vi "Find One Cycle.vi"(11 "data in":u16[][](array[numeric])) -> (1 "n crossings":u16, 3 "data out":u16[][](array[numeric]))   [LabVIEW 2018]
panel:
  out "loop iterations":i32
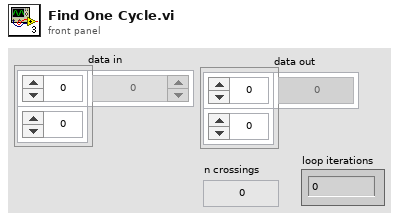
[diagram p1: front panel]
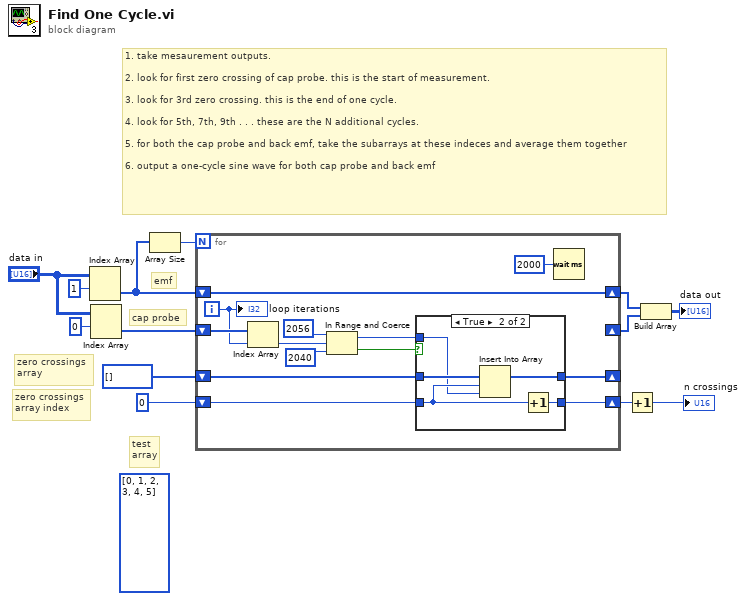
[diagram p0: block diagram]
diagram:
  (unwired) u16[] [0, 1, 2, 3, 4, 5] ("data in")
  # "test\narray"
  # "cap probe"
  # "emf"
  # "zero crossings\narray index"
  # "zero crossings\narray"
  # "1. take mesaurement outputs.\n\n2. look for first zero crossing of cap probe. this is the start of measurement.\n\n3. look for 3rd zero crossing. this is the end of one cycle.\n\n4. look for 5th, 7th, 9th . . . these are the N additional cycles.\n\n5. for both the cap probe and back emf, take the subarrays at these indeces and average them together\n\n6. output a one-cycle sine wave for both cap probe and back emf"
  n1 = Index Array(array="data in", index (row)=1) -> (element=w5:u16[])  [unwired: 1 in]
  n2 = Index Array(array="data in", index (row)=0) -> (element=w9:u16[])  [unwired: 1 in]
  n3 = Array Size(array=w5) -> (size(s)=w7:i32)
  n4 = for {
    N: w7 -> [_]
    shift-right: [_] -> w12
    shift-left: w9 -> [w22]
    shift-right: [w23] -> w6
    shift-left: w5 -> [w23]
    shift-right: [w14] -> _
    shift-left: u16[] [] ("subarray") -> [w17]
    shift-right: [w15] -> w2
    shift-left: u16 0 ("n cycles") -> [w16]
    i -> [w20]
    n5 = Index Array(array=w22, index=w20) -> (element=w21:u16)
    n6 = In Range and Coerce(upper limit=u16 2056, x=w21, lower limit=u16 2040) -> (coerced(x)=w18:u16, In Range?=w19:bool)
    n7 = case shown="True" w19 {
      tunnel: w18 -> [_ w29]
      tunnel: w17 -> [w27 w32]
      tunnel: w16 -> [w28 w31]
      tunnel: [w28 w33] -> w15
      tunnel: [w27 w30] -> w14
      frame False {
      }
      frame True {
        n8 = Insert Into Array(array=w32, index=w31, new element=w29) -> (w30:u16[])
        n9 = Increment(x=w31) -> (x+1=w33:u16)
      }
    }
    n10 = Wait (ms)(milliseconds to wait=u32 2000) -> ()  [unwired: 1 out]
    "loop iterations" <- w20
  }
  n11 = Increment(x=w2) -> (x+1=→"n crossings":u16)
  n12 = Build Array(w6, w12) -> (→"data out":u16[][])
